vi "Spectrometer - ParseUnits.vi"(10 "String Array":string[](array[string])) -> (0 "Y Axis Unit":string, 1 "Y Axis Name":string, 2 "X Axis Unit":string, 3 "X Axis Name":string, 4 "Y Unit (ring)":i32, 6 "X Unit (ring)":i32)   [LabVIEW 2014]
panel:
  # "LICENSED MATERIALS – PROPERTY OF IBM\nCopyright IBM Corp. 2016,\nALL RIGHTS RESERVED"
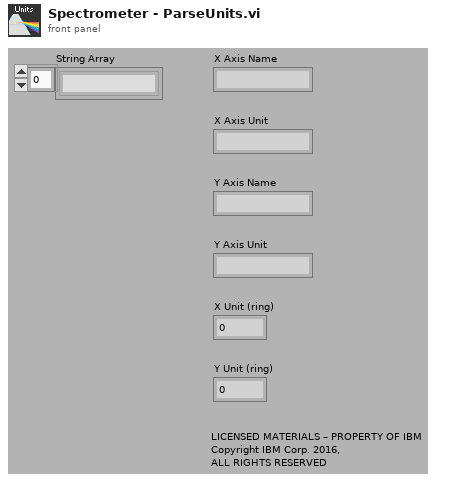
[diagram p1: front panel]
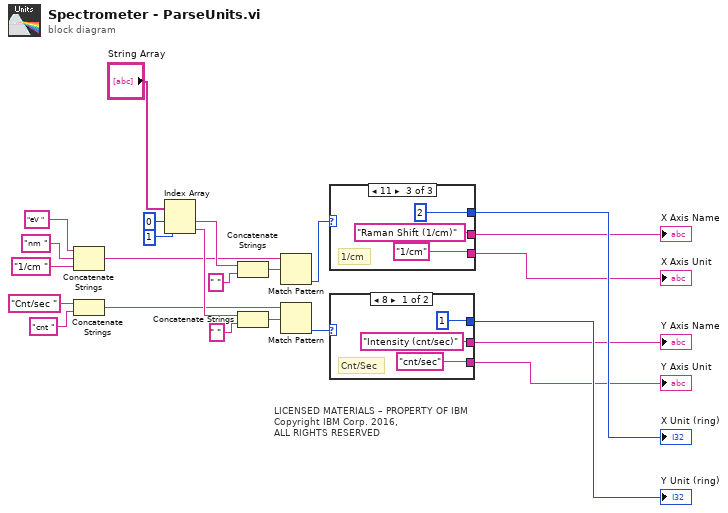
[diagram p0: block diagram]
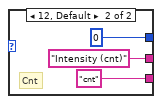
[diagram p2: hidden frame]
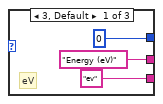
[diagram p3: hidden frame]
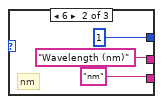
[diagram p4: hidden frame]
diagram:
  # "LICENSED MATERIALS – PROPERTY OF IBM\nCopyright IBM Corp. 2016,\nALL RIGHTS RESERVED"
  n1 = Concatenate Strings("eV ", "nm ", "1/cm ") -> (w9:string)
  n2 = Concatenate Strings("Cnt/sec ", "cnt ") -> (w10:string)
  n3 = Index Array(array="String Array", index #1=0 ("index"), index #2=1 ("index")) -> (element #1=w11:string, element #2=w16:string)
  n4 = Concatenate Strings(w11, " ") -> (w15:string)
  n5 = Concatenate Strings(w16, " ") -> (w14:string)
  n6 = Match Pattern(string=w9, regular expression=w15) -> (offset past match=w17:i32)  [unwired: 4 out]
  n7 = Match Pattern(string=w10, regular expression=w14) -> (offset past match=w18:i32)  [unwired: 4 out]
  n8 = case shown="11" w17 {
    tunnel: [u16 0 ("Value") u16 1 ("Value") u16 2 ("Value")] -> w23
    tunnel: ["Energy (eV)" "Wavelength (nm)" "Raman Shift (1/cm)"] -> w19
    tunnel: ["ev" "nm" "1/cm"] -> w20
    frame 3, Default {
      # "eV"
    }
    frame 6 {
      # "nm"
    }
    frame 11 {
      # "1/cm"
    }
  }
  "X Unit (ring)" <- w23
  "X Axis Unit" <- w20
  "X Axis Name" <- w19
  n9 = case shown="8" w18 {
    tunnel: [u16 1 ("Value") u16 0 ("Value")] -> w24
    tunnel: ["Intensity (cnt/sec)" "Intensity (cnt)"] -> w21
    tunnel: ["cnt/sec" "cnt"] -> w22
    frame 8 {
      # "Cnt/Sec"
    }
    frame 12, Default {
      # "Cnt"
    }
  }
  "Y Unit (ring)" <- w24
  "Y Axis Unit" <- w22
  "Y Axis Name" <- w21
